vi "HIOKI PW3390 Continuous Acquisition.vi"() -> ()   [LabVIEW 2009]
doc: "Continues to output the specified measurement data in 100ms cycle."
uses:
  <instrlib>/PW3390/Common/_Initialize/HIOKI PW3390 Initialize LAN.vi
  <instrlib>/PW3390/Common/_Initialize/HIOKI PW3390 Initialize RS-232C.vi
panel:
  out "Selected Item out":string[](array[string])
  out "Data out":dbl[](array[numeric])
  in  "Item":T1(array[cluster])=[{"Item"=enum."Urms", "Ch(0:Ch1)"=enum."1"}, {"Item"=enum."Urms", "Ch(0:Ch1)"=enum."2"}, {"Item"=enum."Urms", "Ch(0:Ch1)"=enum."3"}, {"Item"=enum."Urms", "Ch(0:Ch1)"=enum."4"}]
  out "error out":errorcluster
  in  "Communication Interface":enum16{"LAN", "RS-232C"}(ring)
  in  "COM Port":refnum<visa-resource-name>="COM1"
  in  "baud rate (38400bps)":u32=38400
  in  "IP Address":string="192.168.1.1"
  in  "Stop":bool
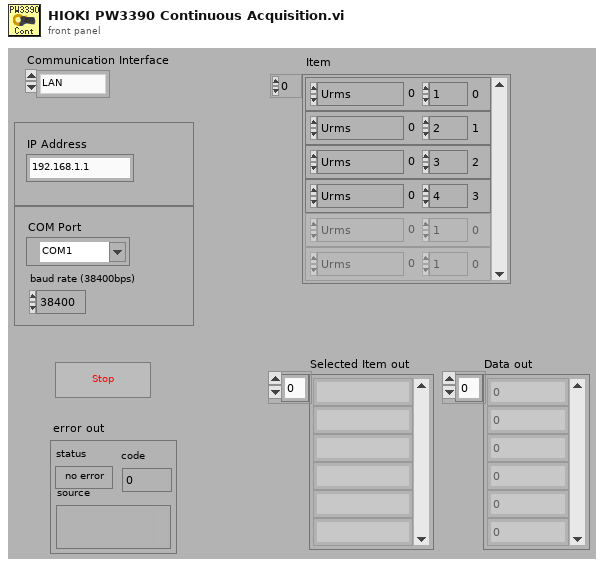
[diagram p1: front panel]
types:
  T1 = cluster{"Item":enum16{"Urms", "Umn", "Uac", "Udc", "Ufnd", "Upk+", "Upk-", "Uthd", "Urf", "Uunb", "Irms", "Imn", "Iac", "Idc", "Ifnd", "Ipk+", "Ipk-", "Ithd", "Irf", "Iunb", "P", "S", "Q", "PF", "DEG U", "DEG I", "DEG P", "f", "EFFI", "LOSS", "IH+", "IH-", "IH", "WP+", "WP-", "WP", "CH A", "CH B", "Pm", "Slip", "Laptime", "Laptime(ms)"}, "Ch(0:Ch1)":enum16{"1", "2", "3", "4", "12", "34", "123"}}[]
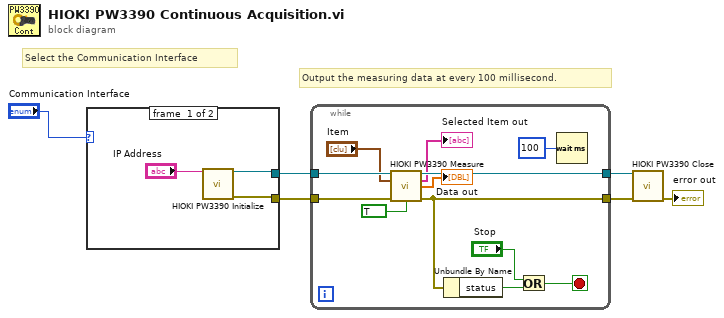
[diagram p0: block diagram]
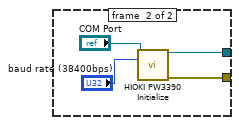
[diagram p2: hidden frame]
diagram:
  # "Select the Communication Interface"
  # "Output the measuring data at every 100 millisecond."
  n1 = case shown="\"LAN\", デフォルト" "Communication Interface" {
    tunnel: [w8 w13] -> w3
    tunnel: [w7 w12] -> w2
    frame #0 {
      n2 = call-poly <instrlib>:"HIOKI PW3390 Initialize.vi"("IP Address"="IP Address") -> ("VISA Resource out"=w8:refnum<visa-resource-name>, "error out"=w7:errorcluster)  [unwired: 12 in, 1 out]
    }
    frame #1 {
      n3 = call-poly <instrlib>:"HIOKI PW3390 Initialize.vi"("COM Port"="COM Port", "baud rate (38400bps)"="baud rate (38400bps)") -> ("VISA Resource out"=w13:refnum<visa-resource-name>, "error out"=w12:errorcluster)  [unwired: 11 in, 1 out]
    }
  }
  n4 = while {
    tunnel: [w25] -> w6
    tunnel: [w21] -> w5
    tunnel: w3 -> [w19]
    tunnel: w2 -> [w18]
    stop <- w22 stop-if-true
    n5 = call <instrlib>:"HIOKI PW3390 Measure.vi"("VISA Resource"=w19, "Item"="Item", "error in (no error)"=w18, "Error Out (F: Off)"=TRUE) -> ("VISA Resource out"=w25:refnum<visa-resource-name>, "Selected Item out"=→"Selected Item out":string[], "Data out"=→"Data out":dbl[], "error out"=w21:errorcluster)  [unwired: 6 in, 2 out]
    n6 = Unbundle By Name(w21) -> ("status"=w20:bool)
    n7 = Or(x="Stop", y=w20) -> (x .or. y?=w22:bool)
    n8 = Wait (ms)(milliseconds to wait=u32 100) -> ()  [unwired: 1 out]
  }
  n9 = call <instrlib>:"HIOKI PW3390 Close.vi"("VISA Resource"=w6, "error in (no error)"=w5) -> ("error out"=→"error out":errorcluster)  [unwired: 13 in]
